vi "Unload OpenCLV DLL.vi"(8 "Error In":errorcluster) -> (0 "Error Out":errorcluster)   [LabVIEW 2012, in "OpenCLV x64.lvlib"]
uses:
  OpenCLV x64.lvlib
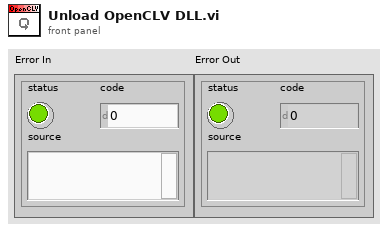
[diagram p1: front panel]
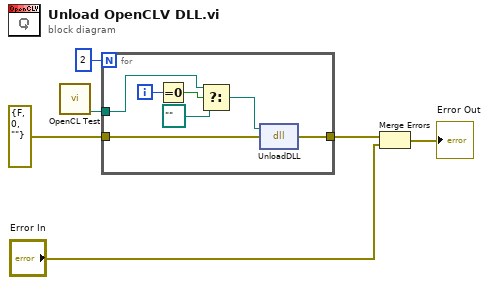
[diagram p0: block diagram]
diagram:
  n1 = call "OpenCL Test.vi"() -> ("DLL To Use"=w1:path)  [unwired: 11 in]
  n2 = for {
    N: 2 -> [_]
    tunnel: errorcluster {"status"=FALSE, "code"=0, "source"=""} ("error IO") -> [w13]
    tunnel: [w12] -> w5
    tunnel: w1 -> [w9]
    i -> [w11]
    n3 = Equal To 0?(x=w11) -> (x = 0?=w10:bool)
    n4 = Select(t=w9, s=w10, f=path "") -> (s? t:f=w7:path)
    n5 = dll-call lib="?" fn="UnloadDLL"(path in=w7, error in=w13) -> (error out=w12:errorcluster)  [unwired: 2 in, 1 out]
  }
  n6 = Merge Errors(w5, "Error In") -> (→"Error Out":errorcluster)
